vi "Inverse Kinematics Solution to Pod Setpoints.vi"(10 "actual theta":dbl, 11 "v + target":cluster{"velocity":dbl, "target theta":dbl}) -> (2 "Substitution Performed?":bool, 3 "new v + travel":cluster{"velocity":dbl, "travel angle":dbl})   [LabVIEW 2025]
doc: "takes the <b>current velocity</b> and <b>wanted target angle</b> to travel, finds the most efficient angle to travel, and outputs the <b>new velocity</b> and the <b>travel angle.</b>\n(used in inverse kinematics)"
uses:
  <vilib>/Analysis/coordinate.llb/Angle Range (Degree).ctl
  <vilib>/Analysis/coordinate.llb/Angle Units.ctl
  <vilib>/Analysis/coordinate.llb/Wrap Angle (scalar).vi
  3d6f3475-1d8e-4577-a545-ae6b5bebe0ce.vi
  <vilib>/Analysis/NI_AAL_Angle.lvlib
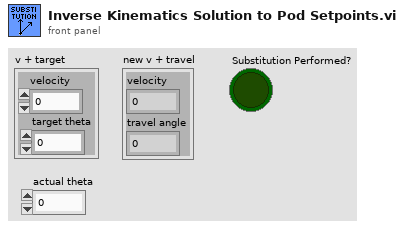
[diagram p1: front panel]
types:
  T1 = typedef "NI_AAL_Angle.lvlib/Angle Units.ctl" = i32
  T2 = typedef "NI_AAL_Angle.lvlib/Angle Range (Degree).ctl" = u16
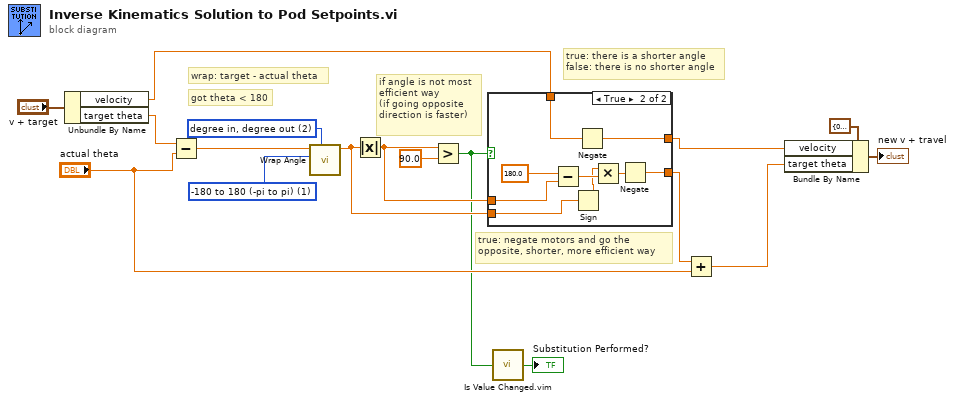
[diagram p0: block diagram]
diagram:
  w16 = T1 2 items=["radian in, radian out", "radian in, degree out", "degree in, degree out", "degree in, radian out"] ("angle units")
  w17 = T2 1 items=["none", "-180 to 180 (-pi to pi)", "0 to 360 (0 to 2pi)"] ("angle range")
  # "true: negate motors and go the\nopposite, shorter, more efficient way"
  # "if angle is not most\nefficient way\n(if going opposite \ndirection is faster)"
  # "true: there is a shorter angle\nfalse: there is no shorter angle"
  # "got theta < 180"
  # "wrap: target - actual theta"
  n1 = Unbundle By Name("v + target") -> ("velocity"=w12:dbl, "target theta"=w14:dbl)
  n2 = Subtract(x=w14, y="actual theta") -> (x-y=w13:dbl)
  n3 = call-poly <vilib>:"Wrap Angle.vi"("angle units"=w16, "angle range"=w17, "angle in"=w13) -> ("angle out"=w8:dbl)  [unwired: 7 in, 1 out]
  n4 = Absolute Value(x=w8) -> (abs(x)=w6:dbl)
  n5 = Greater?(x=w6, y=90.0) -> (0:w2:bool)
  n6 = case shown="True" w2 {
    tunnel: w12 -> [w19 w28]
    tunnel: [w19 w27] -> w11
    tunnel: w6 -> [_ w25]
    tunnel: [w18 w26] -> w7
    tunnel: w8 -> [w18 w22]
    frame False {
    }
    frame True {
      n7 = Subtract(x=180.0, y=w25) -> (x-y=w23:dbl)
      n8 = Sign(1:w22) -> (0:w21:dbl)
      n9 = Negate(x=w28) -> (-x=w27:dbl)
      n10 = Multiply(x=w21, y=w23) -> (x*y=w24:dbl)
      n11 = Negate(x=w24) -> (-x=w26:dbl)
    }
  }
  n12 = call "Is Value Changed.vim"("value"=w2) -> ("changed or first call?"=→"Substitution Performed?":bool)
  n13 = Add(x=w7, y="actual theta") -> (x+y=w4:dbl)
  n14 = Bundle By Name(cluster=cluster{"velocity":dbl, "target theta":dbl} {"velocity"=0.0, "target theta"=0.0}, "velocity"=w11, "target theta"=w4) -> (→"new v + travel":cluster{"velocity":dbl, "target theta":dbl})
